vi "led_piscando.vi"() -> ()   [LabVIEW 2018]
panel:
  in  "stop 3":bool
  out "Boolean 3":bool
  in  "stop 2":bool
  out "Boolean 2":bool
  out "Boolean":bool
  in  "stop":bool
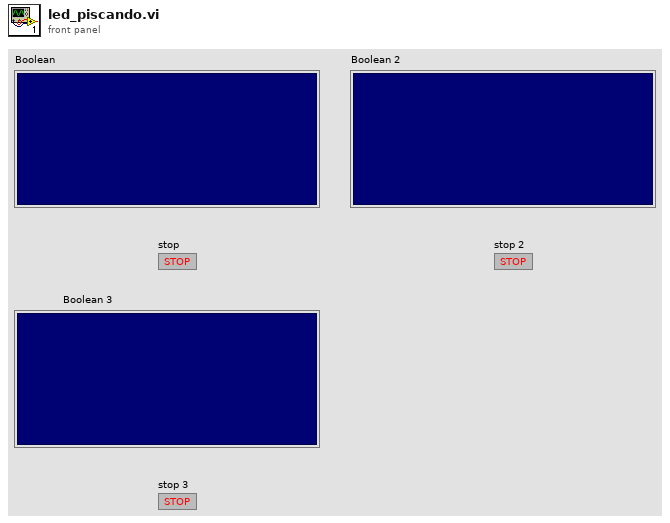
[diagram p1: front panel]
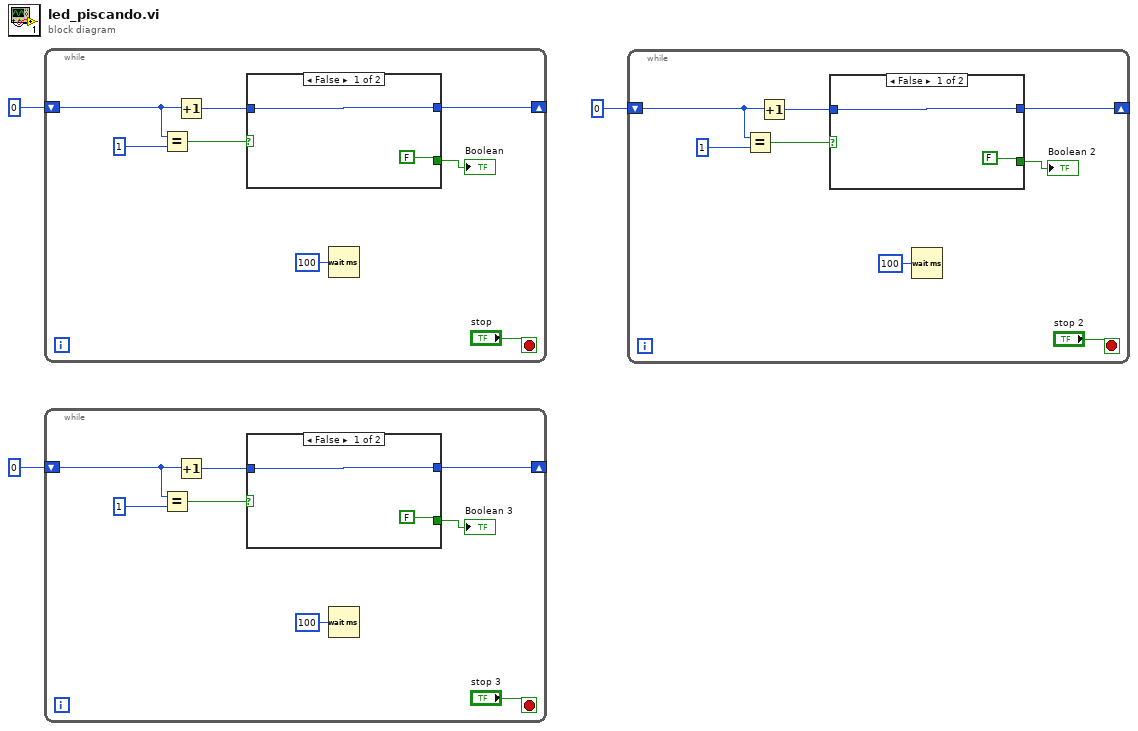
[diagram p0: block diagram]
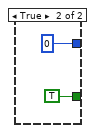
[diagram p2: hidden frame]
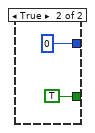
[diagram p3: hidden frame]
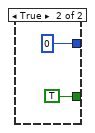
[diagram p4: hidden frame]
diagram:
  n1 = while {
    shift-right: [w8] -> _
    shift-left: 0 -> [w4]
    stop <- "stop" stop-if-true
    n2 = Equal?(x=w4, y=1) -> (x = y?=w9:bool)
    n3 = Increment(x=w4) -> (x+1=w5:i32)
    n4 = case shown="False" w9 {
      tunnel: w5 -> [w13 _]
      tunnel: [w13 0] -> w8
      tunnel: [FALSE TRUE] -> w7
      frame False {
      }
      frame True {
      }
    }
    "Boolean" <- w7
    n5 = Wait (ms)(milliseconds to wait=u32 100) -> ()  [unwired: 1 out]
  }
  n6 = while {
    shift-right: [w20] -> _
    shift-left: 0 -> [w16]
    stop <- "stop 3" stop-if-true
    n7 = Equal?(x=w16, y=1) -> (x = y?=w21:bool)
    n8 = Increment(x=w16) -> (x+1=w17:i32)
    n9 = case shown="False" w21 {
      tunnel: w17 -> [w25 _]
      tunnel: [w25 0] -> w20
      tunnel: [FALSE TRUE] -> w19
      frame False {
      }
      frame True {
      }
    }
    "Boolean 3" <- w19
    n10 = Wait (ms)(milliseconds to wait=u32 100) -> ()  [unwired: 1 out]
  }
  n11 = while {
    shift-right: [w32] -> _
    shift-left: 0 -> [w28]
    stop <- "stop 2" stop-if-true
    n12 = Equal?(x=w28, y=1) -> (x = y?=w33:bool)
    n13 = Increment(x=w28) -> (x+1=w29:i32)
    n14 = case shown="False" w33 {
      tunnel: w29 -> [w37 _]
      tunnel: [w37 0] -> w32
      tunnel: [FALSE TRUE] -> w31
      frame False {
      }
      frame True {
      }
    }
    "Boolean 2" <- w31
    n15 = Wait (ms)(milliseconds to wait=u32 100) -> ()  [unwired: 1 out]
  }
